vi "Read State.vi"(8 "error in (no error)":errorcluster, 11 "Context Actor in":refnum<class "Context Actor.lvclass">) -> (0 "error out":errorcluster, 2 "State":refnum<class "State Pattern.lvclass">, 3 "Context Actor out":refnum<class "Context Actor.lvclass">)   [LabVIEW 2021, in "Context Actor.lvlib" / "Context Actor.lvclass"]
uses:
  Context Actor.lvclass
  Context Actor.lvclass/Context Actor.ctl
  Context State/Context State.lvclass
  C:/PPLs/Design-Patterns/State Pattern/Context Actor/Context State/Context State.lvclass
  C:/PPLs/Design-Patterns/State Pattern/State Pattern/State Pattern.lvclass
  State Pattern/State Pattern.lvclass
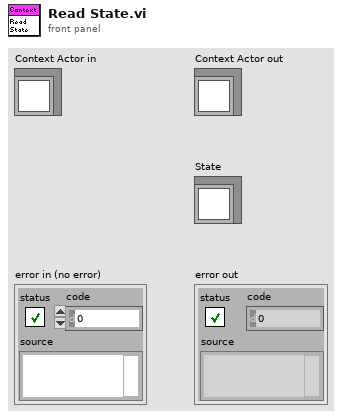
[diagram p1: front panel]
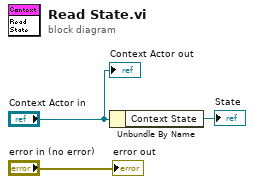
[diagram p0: block diagram]
diagram:
  n1 = Unbundle By Name("Context Actor in") -> ("Context State"=→"State":refnum<class "Context State.lvclass">)
  "error out" <- "error in (no error)"
  "Context Actor out" <- "Context Actor in"
